vi "Flashlamp_Voltage.vi"(8 "error in (no error)":errorcluster, 10 "Voltage (kV)":sgl min=0 max=1.1 step=0.01, 11 "VISA resource name":refnum<visa-resource-name>) -> (0 "error out":errorcluster, 3 "VISA resource name out":refnum<visa-resource-name>)   [LabVIEW 2012, in "Surelite I.lvlib"]
doc: "Resets the instrument and then sends a set of default setup commands to the instrument."
uses:
  Surelite I.lvlib
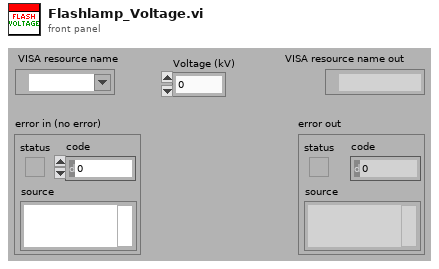
[diagram p1: front panel]
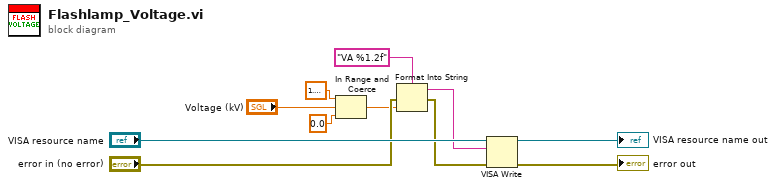
[diagram p0: block diagram]
diagram:
  n1 = In Range and Coerce(upper limit=sgl 1.1, x="Voltage (kV)", lower limit=sgl 0.0) -> (coerced(x)=w3:sgl)  [unwired: 1 out]
  n2 = Format Into String(format string="VA %1.2f", error in="error in (no error)", w3) -> (resulting string=w4:string, error out=w5:errorcluster)  [unwired: 1 in]
  n3 = VISA Write(VISA resource name="VISA resource name", write buffer=w4, error in (no error)=w5) -> (VISA resource name out=→"VISA resource name out":refnum<visa-resource-name>, error out=→"error out":errorcluster)  [unwired: 1 out]
